vi "Rotate Waypoints Pre.vi"(9 "Pt 2":cluster{"x":dbl, "y":dbl, "th":dbl}, 10 "Pt 1":cluster{"x":dbl, "y":dbl, "th":dbl}, 11 "Pt 0":cluster{"x":dbl, "y":dbl, "th":dbl}) -> (1 "Pt 2 out":cluster{dbl, dbl, dbl}, 2 "Pt 1 out":cluster{"Vertex Dist":dbl, dbl, dbl}, 3 "Pt 1 rel to Pt0":cluster{"Vertex Dist":dbl, dbl, dbl})   [LabVIEW 2018]
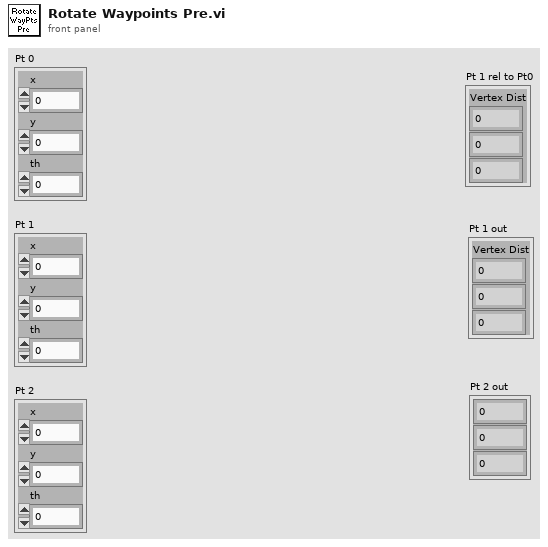
[diagram p1: front panel]
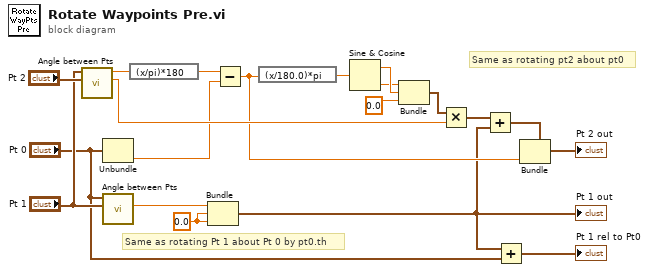
[diagram p0: block diagram]
diagram:
  w9 = 0.0
  # "Same as rotating pt2 about pt0"
  # "Same as rotating Pt 1 about Pt 0 by pt0.th"
  n1 = call "Angle between Pts.vi"("Pt 2"="Pt 2", "Pt 1"="Pt 1") -> ("Distance ft"=w15:dbl, "Angle rad"=w11:dbl)  [unwired: 8 in]
  n2 = Unbundle("Pt 0") -> ("th"=w8:dbl)  [unwired: 2 out]
  n3 = call "Angle between Pts.vi"("Pt 2"="Pt 1", "Pt 1"="Pt 0") -> ("Distance ft"=w4:dbl)  [unwired: 8 in, 1 out]
  n4 = expression code="(x/pi)*180" ("radians to degrees")(w11) -> (w10:dbl)
  n5 = Bundle("Distance ft"=w4, w9, w9) -> (w3:cluster{"Distance ft":dbl, dbl, dbl})  [unwired: 1 in]
  "Pt 1 out" <- w3
  n6 = Subtract(x=w10, y=w8) -> (x-y=w13:dbl)
  n7 = expression code="(x/180.0)*pi" ("degrees to radians")(w13) -> (w20:dbl)
  n8 = Sine & Cosine(0:w20) -> (1:w18:dbl, 2:w17:dbl)
  n9 = Bundle(w17, w18, 0.0) -> (w16:cluster{dbl, dbl, dbl})  [unwired: 1 in]
  n10 = Multiply(x=w16, y=w15) -> (x*y=w7:cluster{dbl, dbl, dbl})
  n11 = Add(x=w7, y=w3) -> (x+y=w6:cluster{dbl, dbl, dbl})
  n12 = Add(x=w3, y="Pt 0") -> (x+y=→"Pt 1 rel to Pt0":cluster{dbl, dbl, dbl})
  n13 = Bundle(cluster=w6, w13) -> (→"Pt 2 out":cluster{dbl, dbl, dbl})  [unwired: 2 in]
